vi "signal input-A.vi"(1 "Reference Signal":cluster{dbl[], dbl[]}, 2 "Coherent Noise":cluster{"F":dbl, "Ampl":dbl}[](array[cluster]), 3 "Time":dbl, 4 "Input":T1 {"AM Frequency" format="%.4f"; "AM Amplitude" format="%.4f"; "LOCK-IN Freq" format="%.2f"; "LOCK-IN Phase" format="%.2f"; "Time Constant (sec)" format="%.2f"; "Low-pass filter slope" format="%.2f"; "Spectral Amplitude" format="%.2f"; "Phase Angle" scale=0.0..360.0 scale format="%.1f"; "Frequency" format="%.2f"; "Amplitude" format="%.2f"}) -> (0 "OUTPUT":T2 {"Input Signal" format="%.2f"; "LOCK-IN Freq" format="%.2f"; "LOCK-IN Phase" format="%.2f"; "Time Constant (sec)" format="%.2f"; "Low-pass filter scope" format="%.2f"; "Time" format="%.2f"; "Spectral Amplitude" format="%.2f"; "Phase Angle" format="%.2f"; "Frequency" format="%.2f"; "Amplitude" format="%.2f"})   [LabVIEW 2011]
doc: "This VI generates the input signal for the Lock-In, starting at TIME. COHERENT NOISE can also be added."
uses:
  <vilib>/ptbypt/NI_PtbyPt.lvlib
panel:
  out "Waveform Chart":cluster{"sine wave":dbl, dbl}(graph)
  out "Signal w/ noise":dbl format="%.2f"
  out "Pure Signal":dbl format="%.2f"
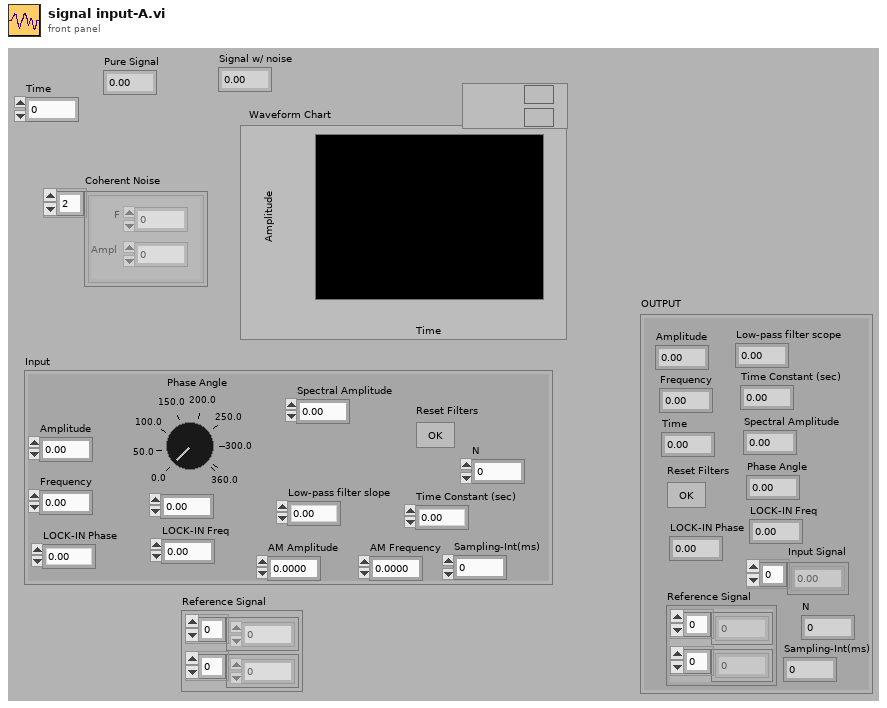
[diagram p1: front panel]
types:
  T1 = cluster{"Amplitude":dbl, "Frequency":dbl, "Phase Angle":dbl, "Spectral Amplitude":dbl, "Low-pass filter slope":dbl, "Time Constant (sec)":dbl, "Reset Filters":bool, "LOCK-IN Phase":dbl, "LOCK-IN Freq":dbl, "AM Amplitude":dbl, "AM Frequency":dbl, "Sampling-Int(ms)":dbl, "N":i32}
  T2 = cluster{"Amplitude":dbl, "Frequency":dbl, "Phase Angle":dbl, "Spectral Amplitude":dbl, "Time":dbl, "Low-pass filter scope":dbl, "Time Constant (sec)":dbl, "Reset Filters":bool, "LOCK-IN Phase":dbl, "LOCK-IN Freq":dbl, "Sampling-Int(ms)":dbl, "Reference Signal":cluster{dbl[], dbl[]}, "Input Signal":dbl[], "N":i32}
  T3 = cluster{"Amplitude":dbl, "Frequency":dbl, "Phase Angle":dbl, "Spectral Amplitude":dbl, "Time":dbl, "Low-pass filter slope":dbl, "Time Constant (sec)":dbl, "Reset Filters":bool, "LOCK-IN Phase":dbl, "LOCK-IN Freq":dbl, "Sampling-Int(ms)":dbl, "Reference Signal":cluster{dbl[], dbl[]}, dbl[], "N":i32}
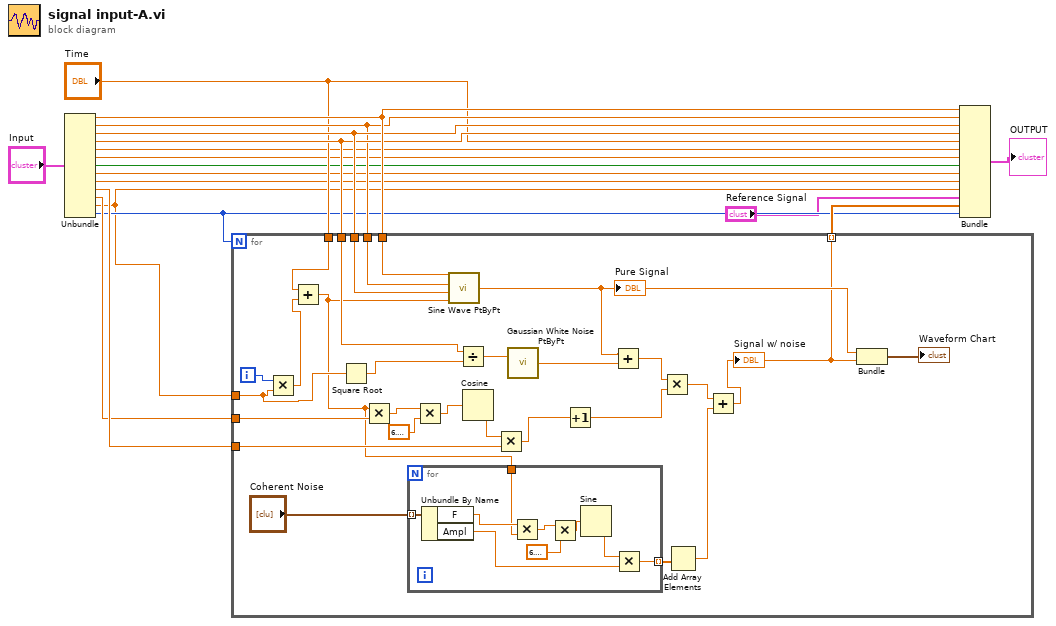
[diagram p0: block diagram]
diagram:
  n1 = Unbundle("Input") -> ("Amplitude"=w18:dbl, "Frequency"=w13:dbl, "Phase Angle"=w17:dbl, "Spectral Amplitude"=w16:dbl, "Low-pass filter slope"=w10:dbl, "Time Constant (sec)"=w9:dbl, "Reset Filters"=w8:bool, "LOCK-IN Phase"=w7:dbl, "LOCK-IN Freq"=w6:dbl, "AM Amplitude"=w5:dbl, "AM Frequency"=w4:dbl, "Sampling-Int(ms)"=w2:dbl, "N"=w3:i32)
  n2 = for {
    N: w3 -> [_]
    tunnel: w18 -> [w46]
    tunnel: w13 -> [w45]
    tunnel: w17 -> [w44]
    tunnel: w16 -> [w29]
    tunnel: "Time" -> [w34]
    tunnel: w4 -> [w41]
    tunnel: w5 -> [w39]
    tunnel: [w23] -> w12 mode=indexing
    tunnel: w2 -> [w31]
    i -> [w35]
    n3 = Multiply(x=w35, y=w31) -> (x*y=w33:dbl)
    n4 = Add(x=w34, y=w33) -> (x+y=w22:dbl)
    n5 = Square Root(x=w31) -> (sqrt(x)=w28:dbl)
    n6 = Multiply(x=w22, y=w41) -> (x*y=w20:dbl)
    n7 = for {
      tunnel: "Coherent Noise" -> [w54] mode=indexing
      tunnel: [w51] -> w26 mode=indexing
      tunnel: w22 -> [w50]
      n8 = Unbundle By Name(w54) -> ("F"=w53:dbl, "Ampl"=w52:dbl)
      n9 = Multiply(x=w53, y=w50) -> (x*y=w49:dbl)
      n10 = Multiply(x=w49, y=6.283185307179586) -> (x*y=w47:dbl)
      n11 = Sine(x=w47) -> (sin(x)=w55:dbl)
      n12 = Multiply(x=w55, y=w52) -> (x*y=w51:dbl)
    }
    n13 = Multiply(x=w20, y=6.283185307179586) -> (x*y=w19:dbl)
    n14 = call <vilib>:"Sine Wave PtByPt.vi"("time"=w22, "phase"=w44, "frequency"=w45, "amplitude"=w46) -> ("sine wave"=w36:dbl)
    "Pure Signal" <- w36
    n15 = Divide(x=w29, y=w28) -> (x/y=w30:dbl)
    n16 = Cosine(x=w19) -> (cos(x)=w40:dbl)
    n17 = Multiply(x=w40, y=w39) -> (x*y=w38:dbl)
    n18 = call <vilib>:"Gaussian White Noise PtByPt.vi"("standard deviation"=w30) -> ("Gaussian white noise"=w43:dbl)  [unwired: 2 in]
    n19 = Increment(x=w38) -> (x+1=w37:dbl)
    n20 = Add(x=w36, y=w43) -> (x+y=w42:dbl)
    n21 = Multiply(x=w42, y=w37) -> (x*y=w24:dbl)
    n22 = Add Array Elements(numeric array=w26) -> (sum=w25:dbl)
    n23 = Add(x=w24, y=w25) -> (x+y=w23:dbl)
    "Signal w/ noise" <- w23
    n24 = Bundle("sine wave"=w36, w23) -> (→"Waveform Chart":cluster{"sine wave":dbl, dbl})  [unwired: 1 in]
  }
  n25 = Bundle("Amplitude"=w18, "Frequency"=w13, "Phase Angle"=w17, "Spectral Amplitude"=w16, "Time"="Time", "Low-pass filter slope"=w10, "Time Constant (sec)"=w9, "Reset Filters"=w8, "LOCK-IN Phase"=w7, "LOCK-IN Freq"=w6, "Sampling-Int(ms)"=w2, "Reference Signal"="Reference Signal", w12, "N"=w3) -> (→"OUTPUT":T3)  [unwired: 1 in]
